vi "Units Matcher - 21032016.vi"(3 "Math-w/-ch-VarID":string[](array[string]), 4 "Comp IDs":string[](array[string]), 5 "OnlySubstanceUnits":string[](array[string]), 6 "Sp_Id_Arr":string[](array[string]), 7 "Kinetic Laws":string[](array[string])) -> (0 "Math-w/-ch-VarID Output":string[](array[string]), 1 "Output Laws":string[](array[string]))   [LabVIEW 2014]
doc: "This VI checks if the flag hasOnlySubstanceUnits is set to \"false\". If it is, it modify the kinetic laws to set the units appropriately for ODE."
uses:
  <vilib>/regexp/Match Regular Expression.xnode
panel:
  out "R-Op":string
  out "L-Op":string
  out "before substring":string
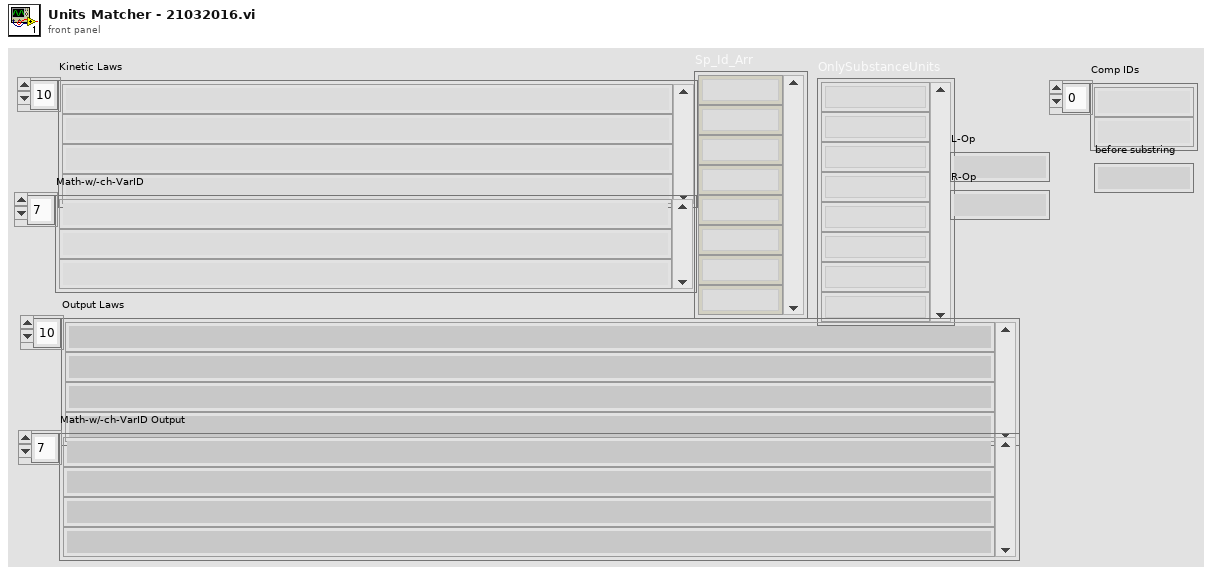
[diagram p1: front panel]
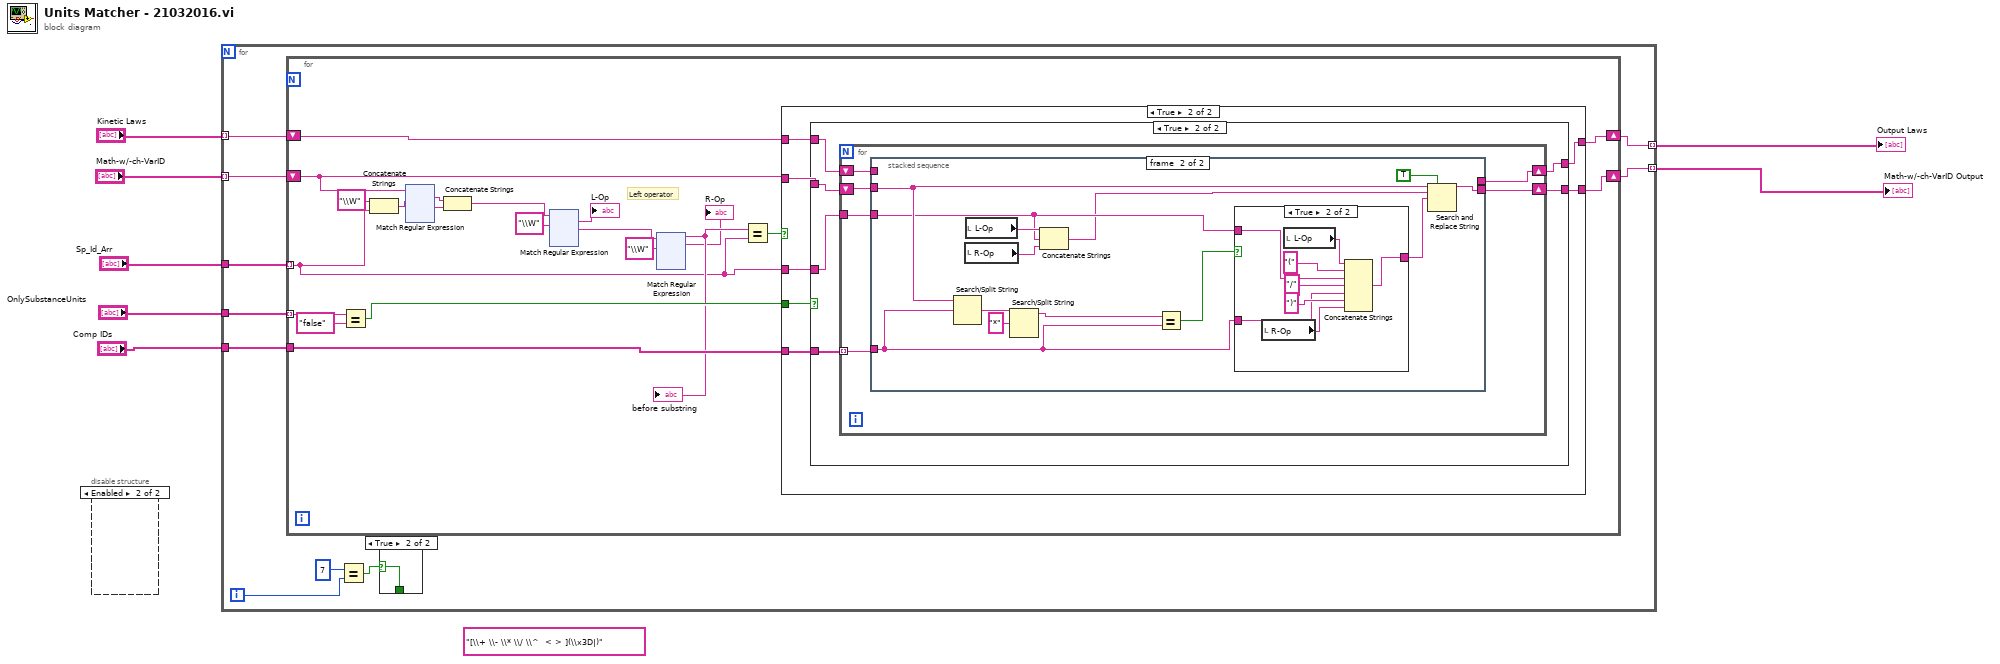
[diagram p0: block diagram]
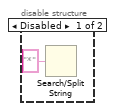
[diagram p2: hidden frame]
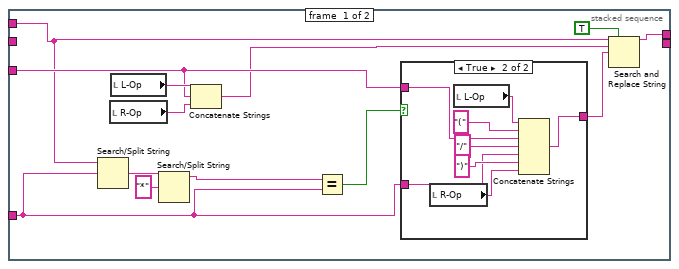
[diagram p6: hidden frame]
diagram:
  (unwired) "[\\+ \\- \\* \\/ \\^  < > ](\\x3D|)" ("Oprts Lst")
  n1 = disable-structure shown="Enabled" {
    frame Disabled {
      n2 = Search/Split String(search string/char (-)="*") -> ()  [unwired: 2 in, 3 out]
    }
    frame Enabled {
    }
  }
  n3 = for {
    tunnel: "Sp_Id_Arr" -> [w18]
    tunnel: "OnlySubstanceUnits" -> [w17]
    tunnel: "Comp IDs" -> [w16]
    tunnel: "Kinetic Laws" -> [w15] mode=indexing
    tunnel: [w14] -> w3 mode=indexing
    tunnel: "Math-w/-ch-VarID" -> [w13] mode=indexing
    tunnel: [w12] -> w1 mode=indexing
    i -> [w9]
    n4 = for {
      tunnel: w18 -> [w29] mode=indexing
      tunnel: w17 -> [w41] mode=indexing
      tunnel: w16 -> [w38]
      shift-right: [w36] -> w14
      shift-left: w15 -> [w37]
      shift-right: [w35] -> w12
      shift-left: w13 -> [w30]
      # "Left operator"
      n5 = Equal?(x=w41, y="false") -> (x = y?=w39:bool)
      n6 = Concatenate Strings("\\W" ("regular expression"), w29) -> (w28:string)
      n7 = xnode "Match Regular Expression"("input string"=w30, "regular expression"=w28) -> ("whole match"=w27:string, "after match"=w26:string)  [unwired: 4 in, 3 out]
      n8 = Concatenate Strings(w27, w26) -> (w24:string)
      n9 = xnode "Match Regular Expression"("input string"=w24, "regular expression"="\\W") -> ("whole match"=→"L-Op":string, "after match"=w23:string)  [unwired: 4 in, 3 out]
      n10 = xnode "Match Regular Expression"("input string"=w23, "regular expression"="\\W") -> ("before match"=w32:string, "whole match"=→"R-Op":string)  [unwired: 4 in, 3 out]
      "before substring" <- w32
      n11 = Equal?(x=w32, y=w29) -> (x = y?=w34:bool)
      n12 = case shown="True" w34 {
        tunnel: w39 -> [_ w392]
        tunnel: w38 -> [_ w391]
        tunnel: w37 -> [w385 w390]
        tunnel: [w385 w389] -> w36
        tunnel: [w384 w388] -> w35
        tunnel: w30 -> [w384 w387]
        tunnel: w29 -> [_ w386]
        frame False {
        }
        frame True {
          n13 = case shown="True" w392 {
            tunnel: w386 -> [_ w400]
            tunnel: w391 -> [_ w399]
            tunnel: w390 -> [w394 w398]
            tunnel: [w394 w397] -> w389
            tunnel: w387 -> [w393 w396]
            tunnel: [w393 w395] -> w388
            frame False {
            }
            frame True {
              n14 = for {
                tunnel: w400 -> [w406]
                tunnel: w399 -> [w404] mode=indexing
                shift-right: [w401] -> w397
                shift-left: w398 -> [w405]
                shift-right: [w402] -> w395
                shift-left: w396 -> [w403]
                n15 = stacked-sequence {
                  tunnel: w406 -> [w410 w431]
                  tunnel: w405 -> [w408 _]
                  tunnel: w404 -> [w414 w436]
                  tunnel: w403 -> [_ w435]
                  tunnel: [_ w429] -> w402
                  tunnel: [w407 _] -> w401
                  frame #0 {
                    n16 = Search/Split String(string=w408, search string/char (-)=w414) -> (match + rest of string=w417:string)  [unwired: 1 in, 2 out]
                    n17 = local read "R-Op"() -> (w411:string)
                    n18 = local read "L-Op"() -> (w412:string)
                    n19 = Search/Split String(string=w417, search string/char (-)="*") -> (substring before match=w416:string)  [unwired: 1 in, 2 out]
                    n20 = Concatenate Strings(w412, w410, w411) -> (w409:string)
                    n21 = Equal?(x=w416, y=w414) -> (x = y?=w415:bool)
                    n22 = case shown="True" w415 {
                      tunnel: w410 -> [w420 w427]
                      tunnel: [w420 w424] -> w418
                      tunnel: w414 -> [_ w423]
                      frame False {
                      }
                      frame True {
                        n23 = local read "R-Op"() -> (w421:string)
                        n24 = local read "L-Op"() -> (w422:string)
                        n25 = Concatenate Strings(w422, "(" ("string"), w427, "/" ("string"), w423, ")" ("string"), w421) -> (w424:string)
                      }
                    }
                    n26 = Search and Replace String(replace all?=TRUE ("replace all? (F)"), input string=w408, search string=w409, replace string=w418) -> (result string=w407:string)  [unwired: 4 in, 3 out]
                  }
                  frame #1 {
                    n27 = Search/Split String(string=w435, search string/char (-)=w436) -> (match + rest of string=w439:string)  [unwired: 1 in, 2 out]
                    n28 = local read "R-Op"() -> (w432:string)
                    n29 = local read "L-Op"() -> (w433:string)
                    n30 = Search/Split String(string=w439, search string/char (-)="*") -> (substring before match=w438:string)  [unwired: 1 in, 2 out]
                    n31 = Concatenate Strings(w433, w431, w432) -> (w430:string)
                    n32 = Equal?(x=w438, y=w436) -> (x = y?=w437:bool)
                    n33 = case shown="True" w437 {
                      tunnel: w431 -> [w442 w449]
                      tunnel: [w442 w446] -> w440
                      tunnel: w436 -> [_ w445]
                      frame False {
                      }
                      frame True {
                        n34 = local read "R-Op"() -> (w443:string)
                        n35 = local read "L-Op"() -> (w444:string)
                        n36 = Concatenate Strings(w444, "(" ("string"), w449, "/" ("string"), w445, ")" ("string"), w443) -> (w446:string)
                      }
                    }
                    n37 = Search and Replace String(replace all?=TRUE ("replace all? (F)"), input string=w435, search string=w430, replace string=w440) -> (result string=w429:string)  [unwired: 4 in, 3 out]
                  }
                }
              }
            }
          }
        }
      }
    }
    n38 = Equal?(x=7, y=w9) -> (x = y?=w11:bool)
    n39 = case shown="True" w11 {
      selector: w11 -> [w19 w20]
      tunnel: [w19 w20] -> _
      frame False {
      }
      frame True {
      }
    }
  }
  "Output Laws" <- w3
  "Math-w/-ch-VarID Output" <- w1
